vi "Lidar Master V5.1.vi"() -> ()   [LabVIEW 2015]
uses:
  Controls/FPGA Nain State.ctl
  <vilib>/Platform/TimedLoop/XDataNode/timing_clust.ctl
  <vilib>/Platform/TimedLoop/XDataNode/nitl_modes.ctl
  <vilib>/Platform/TimedLoop/XDataNode/wakeup.ctl
  <vilib>/rvi/Emulation/niFpgaGetClockAttributes.vi
  <vilib>/rvi/Emulation/niFpgaSctlEmulationGetInTimedLoop.vi
  <vilib>/rvi/Emulation/niFpgaEmulationReportErrorSimple.vi
  <vilib>/rvi/eio/common/nirviEmuTemplateMethod_errors.vi
  <vilib>/rvi/Emulation/niFpgaCriticalErrorInLSC.vi
  <vilib>/rvi/Emulation/niFpgaProcessEmulError.vi
  <vilib>/rvi/Memory/Memory_Emulation/nirvimemoryFastEmulation.vi
  <vilib>/rvi/Memory/Memory_Emulation/nirvimemoryEmulation.vi
  <vilib>/rvi/Emulation/niFpgaEmulationIsFPGAContextNoSignature.vi
  <vilib>/rvi/DataTransferAndStorage/Container/Common/niFpgaContainerGetUniqueNameForEmu.vi
  <vilib>/rvi/errors/nirviReportUnexpectedCaseInternalError (U32).vi
  <vilib>/rvi/errors/niFpgaSetErrorForExecOnDevCompSimple.vi
  <vilib>/rvi/eio/common/nirviEmuReportErrorAndStop.vi
  <vilib>/rvi/FIFO/Fifo_Resource/nirvififoEmulationSetSize.vi
  <vilib>/rvi/FIFO/Fifo_Resource/nirviFifoEmulationQueueMgr.vi
  <instcachedir>/0/nirviFifoEmulationQueueMgr_E5CAEC123FF24DC58D834DCA3CDAA9B5.lvgen/nirviFifoEmulationQueueMgr_E5CAEC123FF24DC58D834DCA3CDAA9B5_003.vi
  <vilib>/Utility/error.llb/Clear Errors.vi
  <vilib>/rvi/FIFO/Fifo_Resource/nirvififoEmulationCreateLock.vi
  <vilib>/rvi/FIFO/Fifo_Resource/nirvififoEmulationObtainLock.vi
  <vilib>/rvi/FIFO/Fifo_Resource/nirvififoEmulationReleaseLock.vi
  <vilib>/rvi/occurrence/nirviWaitOnOccurrenceBase.vi
  <vilib>/rvi/errors/nirviReportUnexpectedCaseInternalError.vi
  <vilib>/eio/EIONode/EIONode.xnode
  <vilib>/Platform/TimedLoop/XDataNode/XDataNode.xnode
  <vilib>/rvi/DataTransferAndStorage/Container/XNode/niFpgaContainer.xnode
  <vilib>/rvi/FIFO/Fifo_Resource/nirvififoEmulationRead.vi
  <vilib>/eio/EIOMethodNode/EIOMethodNode.xnode
  <vilib>/Platform/TimedLoop/XDataNode/XDNodeRunTimeDep.lvlib
  LIDAR V2 Globals.vi
panel:
  in  "User Command Commit":bool
  in  "User Command":u8
  in  "User Data 1":u8
  in  "User Data 0":u8
  in  "StartSyncLoop":bool
  out "Trig1":bool
  in  "SendDebugVal":bool
  in  "WriteSenseData":i16
  in  "WriteSensAdd":i16
  in  "WriteSensDataEn":bool
  in  "ActiveSensDeb":u8
  in  "SensScanDeb":bool
  in  "SensorMap":u8[](array[numeric])=[0, 0, 0, 0, 0, 0, 0, 0, 0, 0, 0, 0, 1, 1, 1, 1, 1, 1, 1, 1, 1, 1, 1, 1, 0, 0, 0, 0, 0, 0, 0, 0, 0, 0, 0, 0, 1, 1, 1, 1, 1, 1, 1, 1, 1, 1, 1, 1, 2, 2, 2, 2, 2, 2, 2, 2, 2, 2, 2, 2, 3, 3, 3, 3, 3, 3, 3, 3, 3, 3, 3, 3, 2, 2, 2, 2, 2, 2, 2, 2, 2, 2, 2, 2, 3, 3, 3, 3, 3, 3, 3, 3, 3, 3, 3, 3]
  in  "AiNoOfSamples":u16
  out "User Command Idle":bool
  out "User Command Status":u8
  out "User Error":bool
  out "Configured?":bool
  out "PLL Locked":bool
  in  "SendAiCMD":u16
  in  "NoOfSamples":u16=1247
  in  "DOActivate":u16=10
  in  "PulseEnd":u16=25
  in  "VgaAdd":u32
  in  "VgaData":i16
  in  "FillVga":bool
  in  "PowerBit0":bool
  in  "PowerBit1":bool
  in  "ActiveLedIndexDeb":u16
  in  "LedScanDebEn":bool
  out "Port0":u8=2 format="%.0b"
  out "Port1Bit4":bool
  out "Port1Bit5":bool
  out "Port1":u8 format="%.0b"
  in  "ScanMode":bool
  out "PulseIndex":i16=88
  in  "StartAcq":u16=26
  in  "StartPulse":u16=20
  in  "StartES":u16=15
  in  "StopES":u16=30
  out "EnableSignal":bool
  out "ActiveLedIndex":u16=2
  in  "EndOfPulseGen":bool=TRUE
  in  "SamplingEnable":bool
  in  "SingleFrame":bool
  out "MainState":T1=enum."ActivatePulseCycle"
  in  "NoOfLeds":u16=95
  in  "PulsePerLed":i16=199
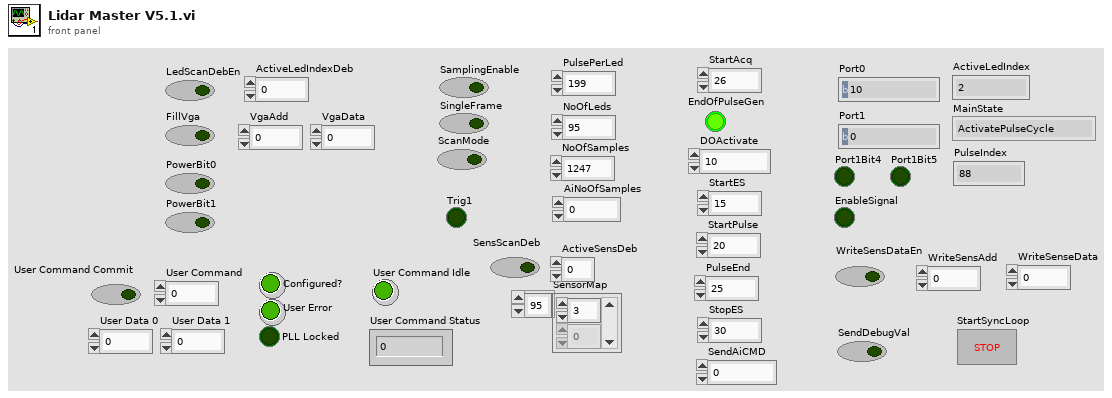
[diagram p1: front panel]
types:
  T1 = typedef "FPGA Nain State.ctl" = enum16{"WaitForStart", "SelectActiveLed", "WaitForNextPulse", "ActivatePulseCycle", "Error"}
  T2 = typedef "XDNodeRunTimeDep.lvlib/timing_clust.ctl" = cluster{"Expected End [f-1]":u64, "Actual End [f-1]":u64, "Finished Late? [f-1]":bool, "Expected End [i-1]":u64, "Actual End [i-1]":u64, "Finished Late? [i-1]":bool, "Expected Start [i]":u64, "Actual Start [i]":u64, "Expected Start [f]":u64, "Actual Start [f]":u64, "Source Name":string, "Structure Name":string, "Period":i64, "Deadline":i64, "Offset":i64, "Start":i64, "Priority":i32, "Timeout":i32, "Mode":T3, "Wakeup Reason":T4, "Error":errorcluster, "Source Type":string, "Secondary Source Type":string, "Global End Time":u64, "Global Start Time":u64, "Frame Duration":u64, "Iteration Duration":u64, "Assigned CPU":i32, "I/O Scan Engine Mode":u32}
  T3 = typedef "XDNodeRunTimeDep.lvlib/nitl_modes.ctl" = enum32{"No Change", "Process missed periods, maintain original phase", "Discard missed periods, maintain original phase", "Process missed periods, ignore original phase", "Discard missed periods, ignore original phase"}
  T4 = typedef "XDNodeRunTimeDep.lvlib/wakeup.ctl" = enum32{"Normal", "Aborted", "Asynchronous wakeup", "Timing source error", "Timed loop error", "Timeout"}
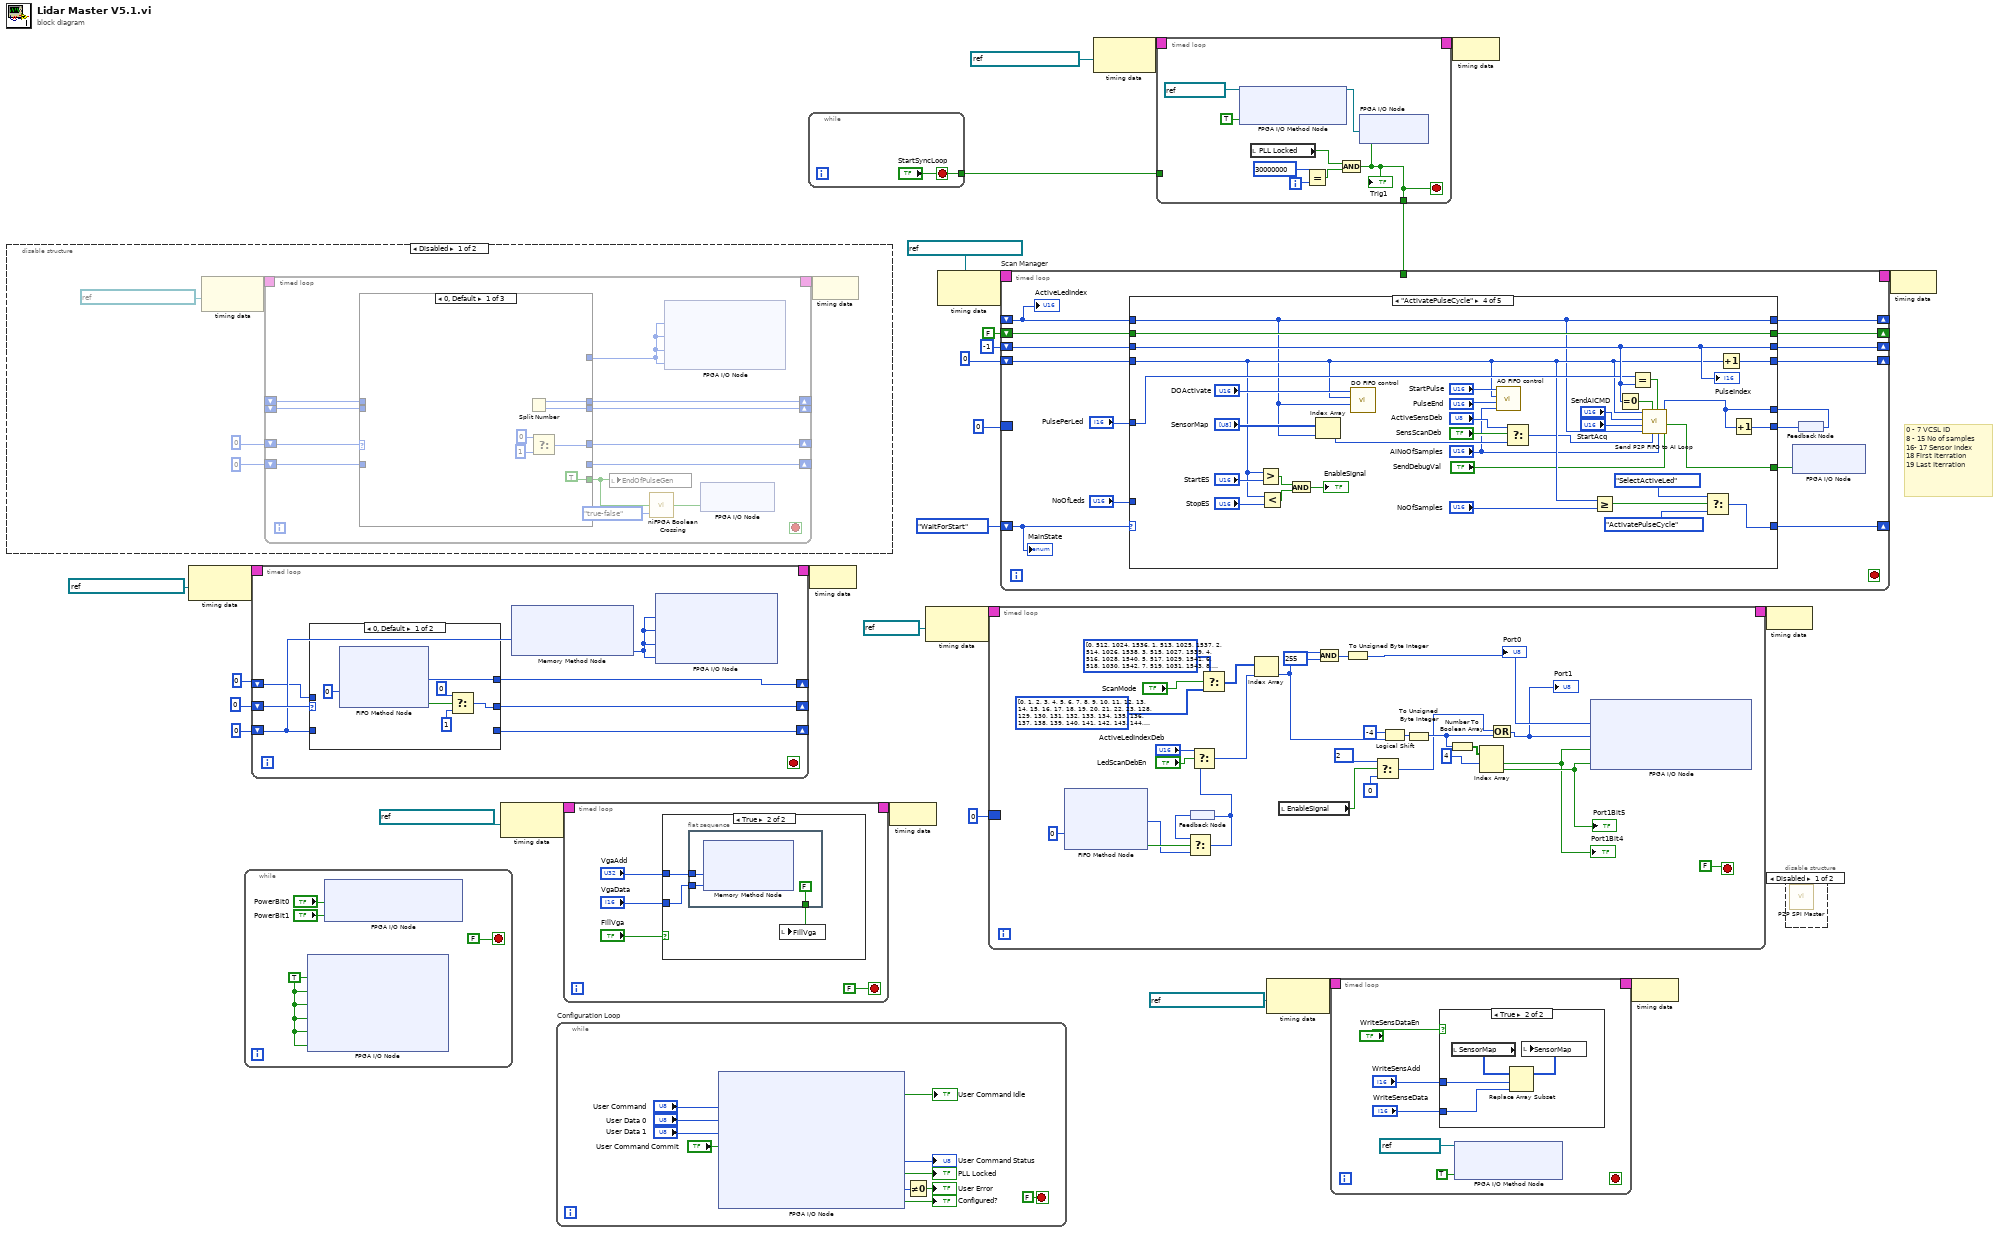
[diagram p0: block diagram]
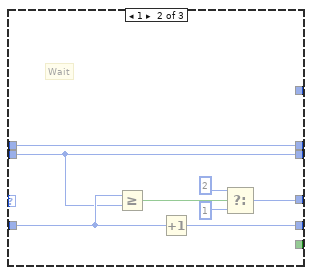
[diagram p4: hidden frame]
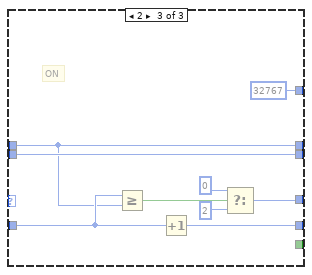
[diagram p5: hidden frame]
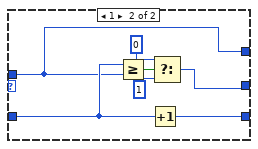
[diagram p7: hidden frame]
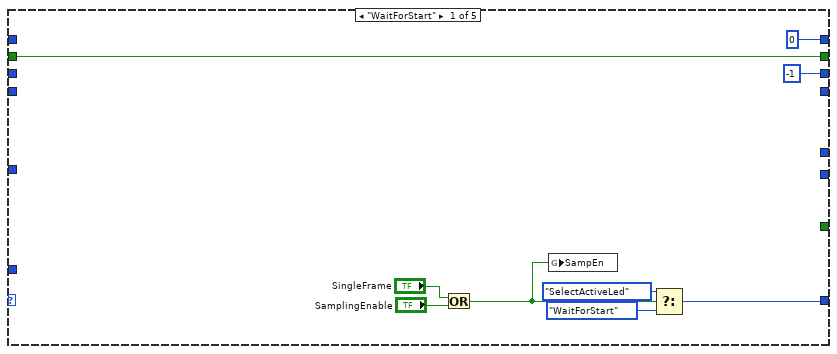
[diagram p9: hidden frame]
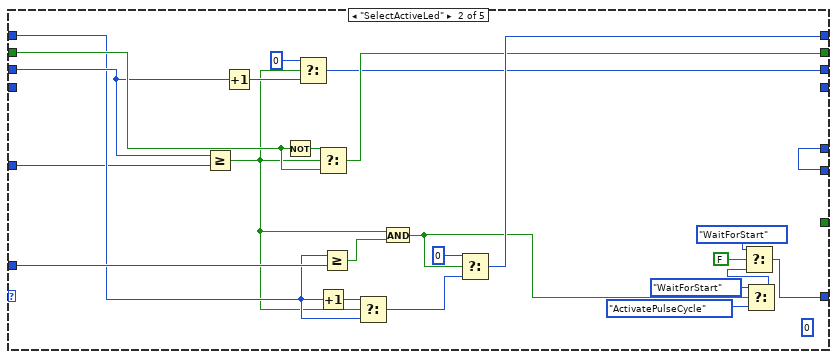
[diagram p10: hidden frame]
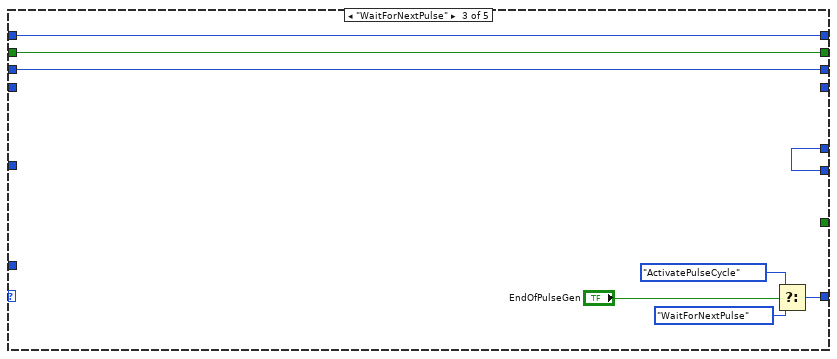
[diagram p11: hidden frame]
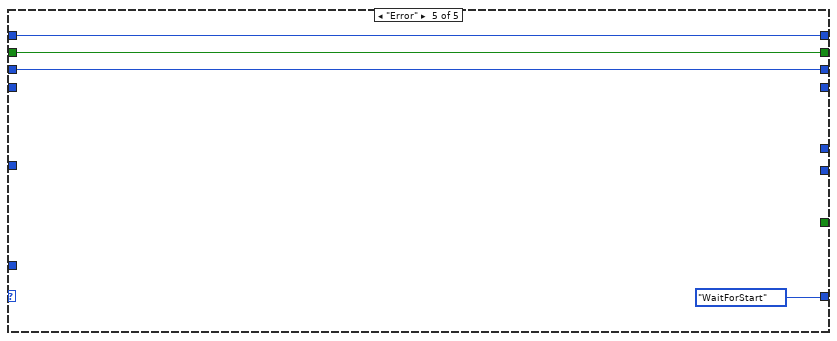
[diagram p12: hidden frame]
diagram:
  # "0 - 7 VCSL ID\n8 - 15 No of samples\n16- 17 Sensor index\n18 First Iterration\n19 Last Iterration"
  n1 = disable-structure shown="Disabled" {
    frame Disabled {
      n2 = node-c288(refnum<k21> "IO Module\\Data Clock" ("Source Name")) -> (w34:T2)
      n3 = timed-loop {
        timing: w34 -> [_]
        timing-out: [_] -> w33
        shift-right: [w45] -> _
        shift-left: i16 0 -> [w46]
        shift-right: [w44] -> _
        shift-left: u32 0 -> [w38]
        shift-right: [w43] -> _
        shift-left: _ -> [w41]
        shift-right: [w42] -> _
        shift-left: _ -> [w40]
        stop <- _ stop-if-true
        n4 = case shown="0, Default" w46 {
          tunnel: [w51 w59 w68] -> w45
          tunnel: [_ w61 w70] -> w44
          tunnel: w38 -> [_ w60 w69]
          tunnel: [w49 w57 w66] -> w43
          tunnel: [w48 w54 w63] -> w42
          tunnel: w41 -> [_ w57 w66]
          tunnel: w40 -> [_ w54 w63]
          tunnel: [_ _ i16 32767 ("IO Module\\AO 0 N")] -> w39
          tunnel: [TRUE _ _] -> w37
          frame 0, Default {
            n5 = Split Number() -> (hi(x)=w48:u16, lo(x)=w49:u16)  [unwired: 1 in]
            n6 = Select(t=i16 0, f=i16 1) -> (s=w53:bool, s? t:f=w51:i16)
          }
          frame 1 {
            # "Wait"
            n7 = Greater Or Equal?(x=w60, y=w57) -> (x >= y?=w58:bool)
            n8 = Increment(x=w60) -> (x+1=w61:u32)
            n9 = Select(t=i16 2, s=w58, f=i16 1) -> (s? t:f=w59:i16)
          }
          frame 2 {
            # "ON"
            n10 = Greater Or Equal?(x=w69, y=w63) -> (x >= y?=w67:bool)
            n11 = Increment(x=w69) -> (x+1=w70:u32)
            n12 = Select(t=i16 0, s=w67, f=i16 2) -> (s? t:f=w68:i16)
          }
        }
        n13 = local write "EndOfPulseGen"(w37) -> ()
        n14 = call <vilib>:"niFPGA Boolean Crossing.vi"("input"=w37, "direction"=enum8{"either", "false-true", "true-false"}."true-false") -> ("crossing"=w35:bool)  [unwired: 7 in]
        n15 = xnode "FPGA I/O Node"("IO Module\\AO 0 N-3"=w39, "IO Module\\AO 0 N-2"=w39, "IO Module\\AO 0 N-1"=w39, "IO Module\\AO 0 N"=w39) -> ()  [unwired: 4 in, 4 out]
        n16 = xnode "FPGA I/O Node"("PXI_Trig0"=w35) -> ()  [unwired: 1 in, 1 out]
      }
      n17 = node-c288(w33) -> ()
    }
    frame Enabled {
    }
  }
  n18 = node-c288(refnum<k21> "IO Module\\Data Clock" ("Source Name")) -> (w16:T2)
  n19 = while {
    stop <- FALSE stop-if-true
    w77 = TRUE ("IO Module\\PFI 0 WE")
    n20 = xnode "FPGA I/O Node"("IO Module\\PFI 0 WE"=w77, "IO Module\\PFI 1 WE"=w77, "IO Module\\PFI 2 WE"=w77, "IO Module\\PFI 3 WE"=w77, "IO Module\\DIO Port 0 WE"=w77, "IO Module\\DIO Port 1 WE"=w77) -> ()  [unwired: 6 in, 6 out]
    n21 = xnode "FPGA I/O Node"("IO Module\\PFI 2 Wr Data"="PowerBit0", "IO Module\\PFI 3 Wr Data"="PowerBit1") -> ()  [unwired: 2 in, 2 out]
  }
  n22 = timed-loop {
    timing: w16 -> [_]
    timing-out: [_] -> w15
    shift-right: [w84] -> _
    shift-left: u16 0 -> [w83]
    shift-right: [w85] -> _
    shift-left: u8 0 -> [w86]
    shift-right: [w82] -> _
    shift-left: u16 0 ("Element") -> [w81]
    stop <- _ stop-if-true
    n23 = case shown="0, Default" w86 {
      tunnel: [w89 w95] -> w85
      tunnel: w83 -> [_ w98]
      tunnel: [_ w100] -> w84
      tunnel: w81 -> [_ w94]
      tunnel: [w88 w94] -> w82
      frame 0, Default {
        n24 = xnode ("FIFO Method Node")("Timeout"=0) -> ("Element"=w88:u16, "Timed Out?"=w92:bool)  [unwired: 1 in, 1 out]
        n25 = Select(t=u8 0, s=w92, f=u8 1) -> (s? t:f=w89:u8)
      }
      frame 1 {
        n26 = Greater Or Equal?(x=w98, y=w94) -> (x >= y?=w99:bool)
        n27 = Increment(x=w98) -> (x+1=w100:u16)
        n28 = Select(t=u8 0, s=w99, f=u8 1) -> (s? t:f=w95:u8)
      }
    }
    n29 = xnode ("Memory Method Node")("Address"=w83) -> ("Data"=w87:i16)  [unwired: 1 in, 1 out]
    n30 = xnode "FPGA I/O Node"("IO Module\\AO 1 N-3"=w87, "IO Module\\AO 1 N-2"=w87, "IO Module\\AO 1 N-1"=w87, "IO Module\\AO 1 N"=w87) -> ()  [unwired: 4 in, 4 out]
  }
  n31 = node-c288(refnum<k21> "IO Module\\Data Clock" ("Source Name")) -> (w20:T2)
  n32 = while "Configuration Loop" {
    stop <- FALSE stop-if-true
    n33 = xnode "FPGA I/O Node"("IO Module\\User Command"="User Command", "IO Module\\User Data 0"="User Data 0", "IO Module\\User Data 1"="User Data 1", "IO Module\\User Command Commit"="User Command Commit") -> ("IO Module\\User Command Idle"=→"User Command Idle":bool, "IO Module\\User Command Status"=→"User Command Status":u8, "IO Module\\PLL Locked"=→"PLL Locked":bool, "IO Module\\User Error"=w110:u8, "IO Module\\Initialization Done"=→"Configured?":bool)  [unwired: 9 in, 9 out]
    n34 = Not Equal To 0?(x=w110) -> (x != 0?=→"User Error":bool)
  }
  n35 = timed-loop {
    timing: w20 -> [_]
    timing-out: [_] -> w19
    stop <- FALSE stop-if-true
    n36 = case shown="True" "FillVga" {
      tunnel: "VgaAdd" -> [_ w120]
      tunnel: "VgaData" -> [_ w119]
      frame False {
      }
      frame True {
        n37 = flat-sequence {
          tunnel: w120 -> [w123]
          tunnel: w119 -> [w122]
          tunnel: [FALSE ("FillVga")] -> w118
          frame #0 {
            n38 = xnode ("Memory Method Node")("Address"=w123, "Data"=w122) -> ()  [unwired: 1 in, 1 out]
          }
        }
        n39 = local write "FillVga"(w118) -> ()
      }
    }
  }
  n40 = while {
    tunnel: ["StartSyncLoop"] -> w1
    stop <- "StartSyncLoop" stop-if-true
  }
  n41 = node-c288(w15) -> ()
  n42 = node-c288(w19) -> ()
  n43 = node-c288(refnum<k21> "130MHz" ("Source Name")) -> (w27:T2)
  n44 = node-c288(refnum<k21> "IO Module\\Data Clock" ("Source Name")) -> (w29:T2)
  n45 = timed-loop {
    timing: w27 -> [_]
    timing-out: [_] -> w26
    border: u16 0 ("Element") -> [_]
    stop <- FALSE stop-if-true
    n46 = xnode ("FIFO Method Node")("Timeout"=0) -> ("Element"=w135:u16, "Timed Out?"=w136:bool)  [unwired: 1 in, 1 out]
    n47 = feedback #1() -> (w133:u16)
    n48 = Select(t=w133, s=w136, f=w135) -> (s? t:f=w134:u16)
    n49 = feedback-in #1(w134) -> ()
    n50 = Select(t="ActiveLedIndexDeb", s="LedScanDebEn", f=w134) -> (s? t:f=w144:u16)
    n51 = Select(t=u16[] [0, 512, 1024, 1536, 1, 513, 1025, 1537, 2, 514, 1026, 1538, 3, 515, 1027, 1539, 4, 516, 1028, 1540, 5, 517, 1029, 1541, 6, 518, 1030, 1542, 7, 519, 1031, 1543, 8, 520, 1032, 1544, 9, 521, 1033, 1545, 10, 522, 1034, 1546, 11, 523, 1035, 1547, 12, 524, 1036, 1548, 13, 525, 1037, 1549, 14, 526, 1038, 1550, 15, 527, 1039, 1551, 16, 528, 1040, 1552, 17, 529, 1041, 1553, 18, 530, 1042, 1554, 19, 531, 1043, 1555, 20, 532, 1044, 1556, 21, 533, 1045, 1557, 22, 534, 1046, 1558, 23, 535, 1047, 1559, 0, 0, 0, 0, 0, 0, 0, 0, 0, 0, 0, 0, 0, 0, 0, 0, 0, 0, 0, 0, 0, 0, 0, 0, 0, 0, 0, 0, 0, 0, 0, 0, 0, 0, 0, 0, 0, 0, 0, 0, 0, 0, 0, 0, 0, 0, 0, 0, 0, 0, 0, 0, 0, 0, 0, 0, 0, 0, 0, 0, 0, 0, 0, 0, 0, 0, 0, 0, 0, 0, 0, 0, 0, 0, 0, 0, 0, 0, 0, 0, 0, 0, 0, 0, 0, 0, 0, 0, 0, 0, 0, 0, 0, 0, 0, 0, 0, 0, 0, 0, 0, 0, 0, 0, 0, 0, 0, 0, 0, 0, 0, 0, 0, 0, 0, 0, 0, 0, 0, 0, 0, 0, 0, 0, 0, 0, 0, 0, 0, 0, 0, 0, 0, 0, 0, 0, 0, 0, 0, 0, 0, 0, 0, 0, 0, 0, 0, 0, 0, 0, 0, 0, 0, 0, 0, 0, 0, 0, 0, 0, 0, 0, 0, 0, 0, 0, 0, 0, 0, 0, 0, 0, 0, 0, 0, 0, 0, 0, 0, 0, 0, 0, 0, 0, 0, 0, 0, 0, 0, 0, 0, 0, 0, 0, 0, 0, 0, 0, 0, 0, 0, 0, 0, 0, 0, 0, 0, 0, 0, 0, 0, 0, 0, 0, 0, 0, 0, 0, 0, 0, 0, 0, 0, 0] ("Array"), s="ScanMode", f=u16[] [0, 1, 2, 3, 4, 5, 6, 7, 8, 9, 10, 11, 12, 13, 14, 15, 16, 17, 18, 19, 20, 21, 22, 23, 128, 129, 130, 131, 132, 133, 134, 135, 136, 137, 138, 139, 140, 141, 142, 143, 144, 145, 146, 147, 148, 149, 150, 151, 256, 257, 258, 259, 260, 261, 262, 263, 264, 265, 266, 267, 268, 269, 270, 271, 272, 273, 274, 275, 276, 277, 278, 279, 384, 385, 386, 387, 388, 389, 390, 391, 392, 393, 394, 395, 396, 397, 398, 399, 400, 401, 402, 403, 404, 405, 406, 407, 0, 0, 0, 0, 0, 0, 0, 0, 0, 0, 0, 0, 0, 0, 0, 0, 0, 0, 0, 0, 0, 0, 0, 0, 0, 0, 0, 0, 0, 0, 0, 0, 0, 0, 0, 0, 0, 0, 0, 0, 0, 0, 0, 0, 0, 0, 0, 0, 0, 0, 0, 0, 0, 0, 0, 0, 0, 0, 0, 0, 0, 0, 0, 0, 0, 0, 0, 0, 0, 0, 0, 0, 0, 0, 0, 0, 0, 0, 0, 0, 0, 0, 0, 0, 0, 0, 0, 0, 0, 0, 0, 0, 0, 0, 0, 0, 0, 0, 0, 0, 0, 0, 0, 0, 0, 0, 0, 0, 0, 0, 0, 0, 0, 0, 0, 0, 0, 0, 0, 0, 0, 0, 0, 0, 0, 0, 0, 0, 0, 0, 0, 0, 0, 0, 0, 0, 0, 0, 0, 0, 0, 0, 0, 0, 0, 0, 0, 0, 0, 0, 0, 0, 0, 0, 0, 0, 0, 0, 0, 0, 0, 0, 0, 0, 0, 0, 0, 0, 0, 0, 0, 0, 0, 0, 0, 0, 0, 0, 0, 0, 0, 0, 0, 0, 0, 0, 0, 0, 0, 0, 0, 0, 0, 0, 0, 0, 0, 0, 0, 0, 0, 0, 0, 0, 0, 0, 0, 0, 0, 0, 0, 0, 0, 0, 0, 0, 0, 0, 0, 0, 0, 0, 0, 0] ("Array")) -> (s? t:f=w139:u16[])
    n52 = Index Array(array=w139, index=w144) -> (element=w129:u16)
    n53 = local read "EnableSignal"() -> (w137:bool)
    n54 = And(x=w129, y=u16 255) -> (x .and. y?=w149:u16)
    n55 = To Unsigned Byte Integer(number=w149) -> (unsigned 8bit integer=w147:u8)
    "Port0" <- w147
    n56 = Select(t=u8 2, s=w137, f=u8 0) -> (s? t:f=w128:u8)
    n57 = Logical Shift(y=i16 -4, x=w129) -> (x << y=w148:u16)
    n58 = To Unsigned Byte Integer(number=w148) -> (unsigned 8bit integer=w146:u8)
    n59 = Number To Boolean Array(number=w146) -> (Boolean array=w153:bool[])
    n60 = Index Array(array=w153, index #1=4 ("index")) -> (element #1=w131:bool, element #2=w132:bool)  [unwired: 1 in]
    "Port1Bit4" <- w131
    "Port1Bit5" <- w132
    n61 = Or(x=w128, y=w146) -> (x .or. y?=w145:u8)
    "Port1" <- w145
    n62 = xnode "FPGA I/O Node"("IO Module\\DIO Port 0 Wr Data"=w147, "IO Module\\DIO Port 1 Wr Data"=w145, "IO Module\\PFI 0 Wr Data"=w131, "IO Module\\PFI 1 Wr Data"=w132) -> ()  [unwired: 4 in, 4 out]
  }
  n63 = node-c288(refnum<k21> "PXI Clk10 MHz Clock" ("Source Name")) -> (w5:T2)
  n64 = timed-loop {
    timing: w5 -> [_]
    timing-out: [_] -> w4
    tunnel: [w161] -> w2
    tunnel: w1 -> [_]
    i -> [w165]
    stop <- w161 stop-if-true
    n65 = xnode "FPGA I/O Method Node"("FPGA I/O In"=refnum<k21> "PXI_Trig1", "Enable"=TRUE) -> ("FPGA I/O Out"=w158:refnum<k21>)
    n66 = local read "PLL Locked"() -> (w162:bool)
    n67 = Equal?(x=30000000, y=w165) -> (x = y?=w163:bool)
    n68 = And(x=w162, y=w163) -> (x .and. y?=w161:bool)
    "Trig1" <- w161
    n69 = xnode "FPGA I/O Node"("I/O Item"=w161, "FPGA I/O In"=w158) -> ()  [unwired: 1 out]
  }
  n70 = timed-loop "Scan Manager" {
    timing: w29 -> [_]
    timing-out: [_] -> w28
    shift-right: [w181] -> _
    shift-left: FPGA_Nain_State."WaitForStart" ("MainState") -> [w182]
    shift-right: [w176] -> _
    shift-left: _ -> [w171]
    shift-right: [w178] -> _
    shift-left: FALSE -> [w180]
    shift-right: [w179] -> _
    shift-left: i16 -1 -> [w177]
    shift-right: [w172] -> _
    shift-left: u16 0 -> [w173]
    border: u32 0 -> [_]
    tunnel: w2 -> [_]
    stop <- _ stop-if-true
    n71 = feedback #2() -> (w168:u32)
    n72 = case shown="\"ActivatePulseCycle\"" w182 {
      tunnel: [w189 w212 w219 w253 FPGA_Nain_State."WaitForStart" ("MainState")] -> w181
      tunnel: [u16 0 ("ActiveLedIndex") w208 w218 w232 w260] -> w176
      tunnel: w171 -> [_ w200 w218 w232 w260]
      tunnel: [w186 w207 w223 w252 w259] -> w178
      tunnel: w180 -> [w186 w210 w223 w252 w259]
      tunnel: [i16 -1 ("t") w203 w222 w237 w258] -> w179
      tunnel: w177 -> [_ w206 w222 w237 w258]
      tunnel: "NoOfLeds" -> [_ w202 _ _ _]
      tunnel: "PulsePerLed" -> [_ w193 _ w236 _]
      tunnel: w173 -> [_ _ _ w233 _]
      tunnel: [_ _ _ w251 _] -> w172
      tunnel: [_ _ _ w228 _] -> w170
      tunnel: w168 -> [_ w192 w216 w226 _]
      tunnel: [_ w192 w216 w227 _] -> w169
      frame "WaitForStart" {
        n73 = Or(x="SingleFrame", y="SamplingEnable") -> (x .or. y?=w183:bool)
        n74 = global write "LIDAR V2 Globals.vi" "SampEn"(w183) -> ()
        n75 = Select(t=FPGA_Nain_State."SelectActiveLed" ("MainState"), s=w183, f=FPGA_Nain_State."WaitForStart" ("MainState")) -> (s? t:f=w189:T1)
      }
      frame "SelectActiveLed" {
        (unwired) u8 0
        n76 = Greater Or Equal?(x=w206, y=w193) -> (x >= y?=w195:bool)
        n77 = Increment(x=w206) -> (x+1=w205:i16)
        n78 = Not(x=w210) -> (.not. x?=w209:bool)
        n79 = Select(t=i16 0, s=w195, f=w205) -> (s? t:f=w203:i16)
        n80 = Select(t=w209, s=w195, f=w210) -> (s? t:f=w207:bool)
        n81 = Increment(x=w200) -> (x+1=w198:u16)
        n82 = Greater Or Equal?(x=w200, y=w202) -> (x >= y?=w196:bool)
        n83 = Select(t=w198, s=w195, f=w200) -> (s? t:f=w199:u16)
        n84 = And(x=w195, y=w196) -> (x .and. y?=w194:bool)
        n85 = Select(t=u16 0, s=w194, f=w199) -> (s? t:f=w208:u16)
        n86 = Select(t=FPGA_Nain_State."WaitForStart" ("MainState"), s=w194, f=FPGA_Nain_State."ActivatePulseCycle" ("MainState")) -> (s? t:f=w213:T1)
        n87 = Select(t=FPGA_Nain_State."WaitForStart" ("MainState"), s=FALSE, f=w213) -> (s? t:f=w212:T1)
      }
      frame "WaitForNextPulse" {
        n88 = Select(t=FPGA_Nain_State."ActivatePulseCycle" ("MainState"), s="EndOfPulseGen", f=FPGA_Nain_State."WaitForNextPulse" ("MainState")) -> (s? t:f=w219:T1)
      }
      frame "ActivatePulseCycle" {
        n89 = Greater?(x=w233, y="StartES") -> (0:w246:bool)
        n90 = Less?(x=w233, y="StopES") -> (x < y?=w247:bool)
        n91 = And(x=w246, y=w247) -> (x .and. y?=→"EnableSignal":bool)
        n92 = Index Array(array="SensorMap", index=w232) -> (element=w231:u8)
        n93 = call "DO FIFO control.vi"("PulseData"=w232, "Counter"=w233, "DOActivate"="DOActivate") -> ()  [unwired: 9 in]
        n94 = call "AO FIFO control.vi"("NoOfSamples"="AiNoOfSamples", "PulseEnd"="PulseEnd", "Counter"=w233, "PulseStart"="StartPulse") -> ()  [unwired: 8 in]
        n95 = Select(t="ActiveSensDeb", s="SensScanDeb", f=w231) -> (s? t:f=w230:u8)
        n96 = Greater Or Equal?(x=w233, y="NoOfSamples") -> (x >= y?=w256:bool)
        n97 = Equal To 0?(x=w237) -> (x = 0?=w239:bool)
        n98 = Equal?(x=w236, y=w237) -> (x = y?=w238:bool)
        n99 = call "Send P2P FIFO to AI Loop.vi"("SendDebugVal"="SendDebugVal", "DebugVals"=w226, "NoOfSamples"="AiNoOfSamples", "LastIterration"=w238, "SensorID"=w230, "FirstIterration"=w239, "ActiveLedIndex"=w232, "SendAiTrig"="StartAcq", "SendAiCMD"="SendAiCMD", "TimingCounter"=w233) -> ("Trig"=w228:bool)  [unwired: 1 out]
        n100 = Select(t=FPGA_Nain_State."SelectActiveLed" ("MainState"), s=w256, f=FPGA_Nain_State."ActivatePulseCycle" ("MainState")) -> (s? t:f=w253:T1)
        n101 = Increment(x=w233) -> (x+1=w251:u16)
        n102 = Increment(x=w226) -> (x+1=w227:u32)
        "PulseIndex" <- w237
      }
      frame "Error" {
      }
    }
    n103 = xnode "FPGA I/O Node"("PXI_Trig0"=w170) -> ()  [unwired: 1 in, 1 out]
    n104 = feedback-in #2(w169) -> ()
    "MainState" <- w182
    "ActiveLedIndex" <- w171
  }
  n105 = node-c288(refnum<k21> "IO Module\\Data Clock" ("Source Name")) -> (w9:T2)
  n106 = timed-loop {
    timing: w9 -> [_]
    timing-out: [_] -> w8
    stop <- _ stop-if-true
    n107 = case shown="True" "WriteSensDataEn" {
      tunnel: "WriteSensAdd" -> [_ w269]
      tunnel: "WriteSenseData" -> [_ w268]
      frame False {
      }
      frame True {
        n108 = local read "SensorMap"() -> (w271:u8[])
        n109 = Replace Array Subset(array=w271, new element=w268, index=w269) -> (w270:u8[])
        n110 = local write "SensorMap"(w270) -> ()
      }
    }
    n111 = xnode "FPGA I/O Method Node"("FPGA I/O In"=refnum<k21> "PXI_Trig0", "Enable"=TRUE) -> ()  [unwired: 1 out]
  }
  n112 = node-c288(w4) -> ()
  n113 = node-c288(w8) -> ()
  n114 = node-c288(w26) -> ()
  n115 = disable-structure shown="Disabled" {
    frame Disabled {
      n116 = call "P2P SPI Master.vi"() -> ()  [unwired: 12 in]
    }
    frame Enabled {
    }
  }
  n117 = node-c288(w28) -> ()
